vi "eFGV - Bow and Stern.vi"(6 "Action":T1, 8 "Error In":errorcluster, 11 "Bow and Stern":string[][](array[string])) -> (0 "Error Out":errorcluster, 2 "Event Bow and Stern":refnum<user-event>, 3 "Bow and Stern Out":string[][](array[string]))   [LabVIEW 2020]
uses:
  Control/State - eFGV.ctl
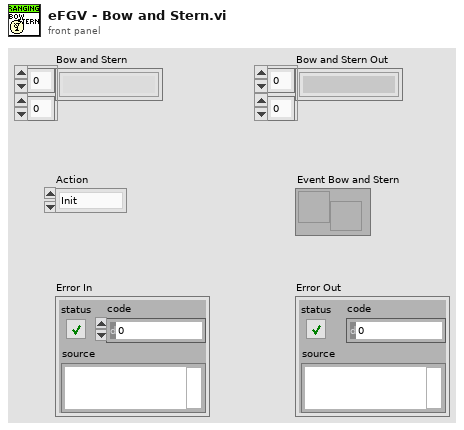
[diagram p1: front panel]
types:
  T1 = typedef "State - eFGV.ctl" = enum16{"Init", "Read", "Write", "Exit"}
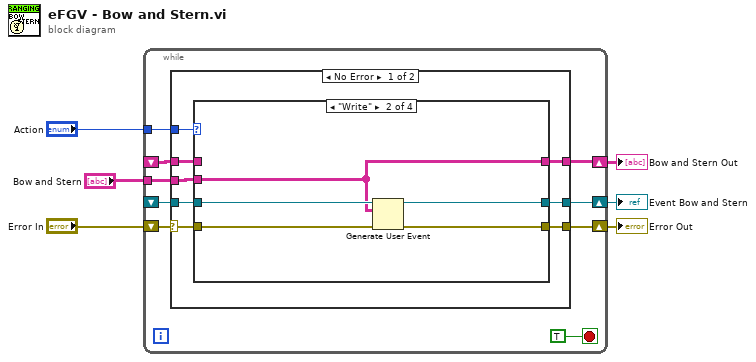
[diagram p0: block diagram]
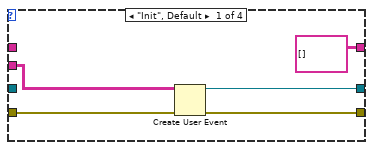
[diagram p2: hidden frame]
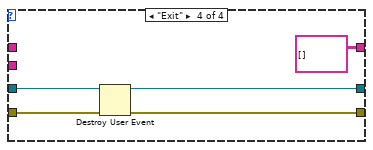
[diagram p4: hidden frame]
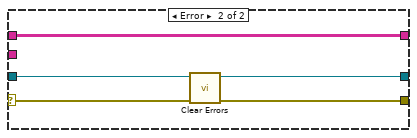
[diagram p5: hidden frame]
diagram:
  n1 = while {
    shift-right: [w14] -> w5
    shift-left: "Error In" -> [w15]
    tunnel: "Action" -> [w13]
    tunnel: "Bow and Stern" -> [w11]
    shift-right: [w10] -> w2
    shift-left: _ -> [w7]
    shift-right: [w9] -> w1
    shift-left: _ -> [w8]
    stop <- TRUE stop-if-true
    n2 = case shown="No Error" w15 {
      selector: w15 -> [w23 w44]
      tunnel: w13 -> [w21 _]
      tunnel: [w22 w43] -> w14
      tunnel: w11 -> [w20 _]
      tunnel: [w19 w41] -> w10
      tunnel: [w18 w42] -> w9
      tunnel: w8 -> [w17 w42]
      tunnel: w7 -> [w16 w41]
      frame No Error {
        n3 = case shown="\"Write\"" w21 {
          tunnel: w23 -> [w28 w33 w36 w40]
          tunnel: [w27 w32 w36 w39] -> w22
          tunnel: w20 -> [w26 w29 _ _]
          tunnel: [string[][] [] ("Bow and Stern") w29 w34 string[][] [] ("Bow and Stern")] -> w19
          tunnel: [w25 w30 w35 w38] -> w18
          tunnel: w17 -> [_ w31 w35 w38]
          tunnel: w16 -> [_ _ w34 _]
          frame "Init", Default {
            n4 = Create User Event(user event datatype=w26, error in=w28) -> (user event=w25:refnum<user-event>, error out=w27:errorcluster)
          }
          frame "Write" {
            n5 = Generate User Event(user event=w31, event data cluster=w29, error in=w33) -> (user event out=w30:refnum<user-event>, error out=w32:errorcluster)  [unwired: 1 in]
          }
          frame "Read" {
          }
          frame "Exit" {
            n6 = Destroy User Event(user event=w38, error in=w40) -> (error out=w39:errorcluster)
          }
        }
      }
      frame Error {
        n7 = call <vilib>:"Clear Errors.vi"("error in (no error)"=w44) -> ("error out"=w43:errorcluster)  [unwired: 5 in, 1 out]
      }
    }
  }
  "Error Out" <- w5
  "Bow and Stern Out" <- w2
  "Event Bow and Stern" <- w1
